vi "Filter Control Drop Event.vi"(8 "error in (no error)":errorcluster, 10 "ControlDropMsg":refnum<class "ControlDropMsg.lvclass">, 11 "Test Executive Builder Event Filter in":refnum<class "Test Executive Builder Event Filter.lvclass">) -> (0 "error out":errorcluster, 1 "Discard?":bool, 3 "Test Executive Builder Event Filter out":refnum<class "Test Executive Builder Event Filter.lvclass">)   [LabVIEW 2017, in "Test Executive Builder Event Filter.lvclass"]
uses:
  Test Executive Builder Event Filter.lvclass
  <vilib>/gpm_packages/@cs/mva-viewable/Source/ActorEvents/IEventAggregator Messages/ControlDropMsg/ControlDropMsg.lvclass
  Test Executive Builder View Messages/Handle Drop Msg/Handle Drop Msg.lvclass
  <vilib>/gpm_packages/@cs/actor-framework-messages/Source/RoundTripMessage/RoundTripMessage.lvclass
  C:/Users/jonmc/Documents/Git/Test Executive Builder/gpm_packages/@cs/actor-framework-messages/Source/RoundTripMessage/RoundTripMessage.lvclass
panel:
  # "No additional\nEvent Data"
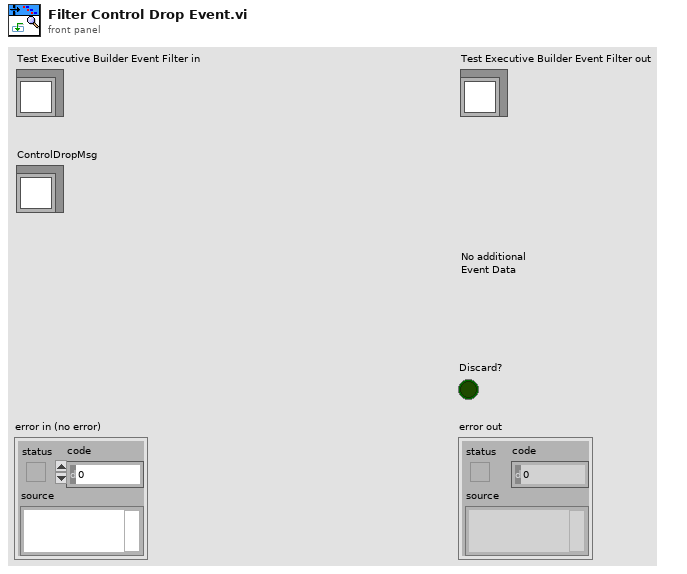
[diagram p1: front panel]
types:
  T1 = typedef "LVPoint32TypeDef.ctl" = cluster{"Horizontal":i32, "Vertical":i32}
  T2 = cluster{"Shift":bool, "Ctrl":bool, "Alt":bool, "Cmd":bool, "Opt":bool}
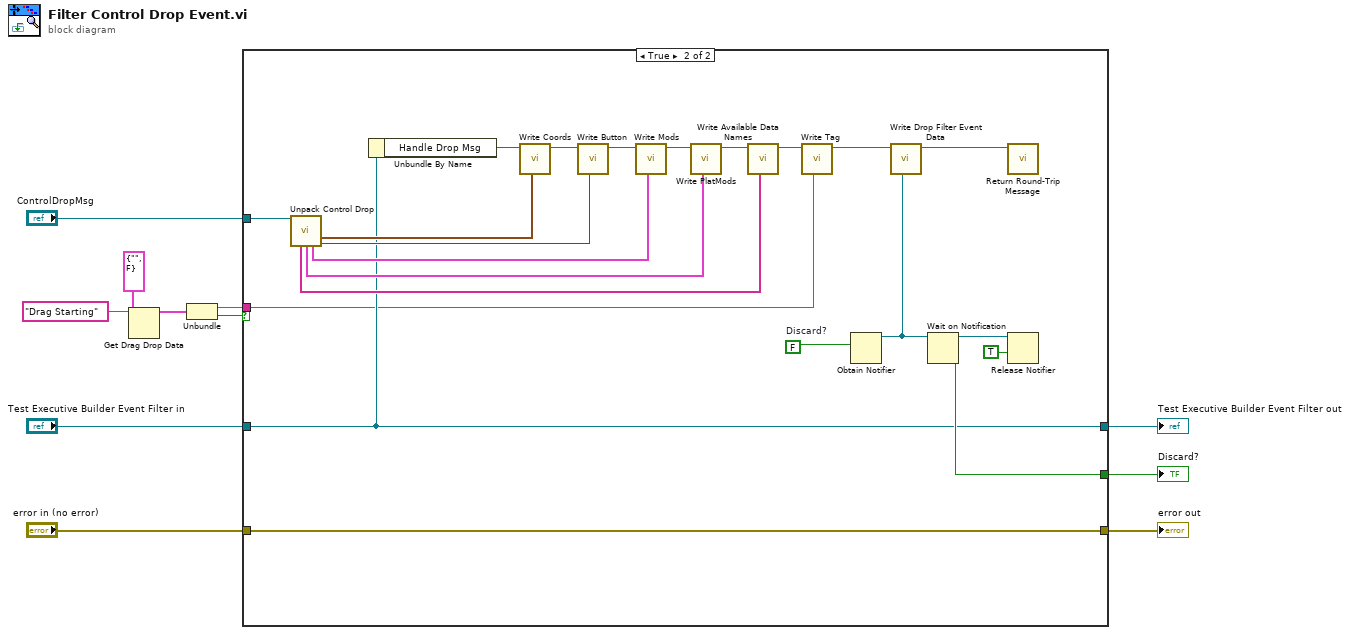
[diagram p0: block diagram]
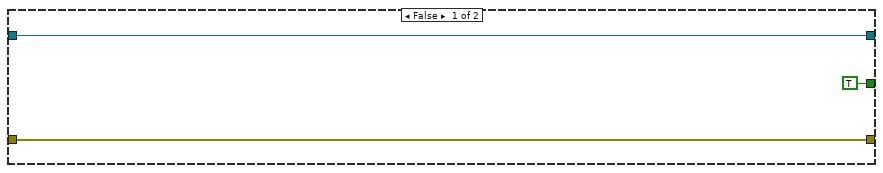
[diagram p2: hidden frame]
diagram:
  n1 = Get Drag Drop Data(8:cluster{"Tag":string, bool} {"Tag"="", FALSE}, 9:"Drag Starting" ("data name")) -> (3:w6:cluster{"Tag":string, bool})  [unwired: 1 in, 1 out]
  n2 = Unbundle(w6) -> ("Tag"=w1:string, w2:bool)
  n3 = case shown="True" w2 {
    tunnel: "ControlDropMsg" -> [_ w36]
    tunnel: [TRUE ("Discard?") w32] -> w10
    tunnel: "Test Executive Builder Event Filter in" -> [w14 w20]
    tunnel: [w14 w20] -> w5
    tunnel: [w12 w19] -> w4
    tunnel: "error in (no error)" -> [w12 w19]
    tunnel: w1 -> [_ w16]
    frame False {
    }
    frame True {
      w34 = FALSE  # Discard?
      n4 = call <vilib>:"Unpack Control Drop.vi"("ControlDropMsg"=w36) -> ("Coords"=w30:T1, "Available Data Names"=w22:string[], "PlatMods"=w24:T2, "Mods"=w26:cluster{"Double Click":bool, "Menu Key":bool}, "Button"=w28:u16)  [unwired: 7 in, 3 out]
      n5 = Unbundle By Name(w20) -> ("Handle Drop Msg"=w31:refnum<class "Handle Drop Msg.lvclass">)
      n6 = call "Write Coords.vi"("Coordinates"=w30, "Handle Drop Msg in"=w31) -> ("Handle Drop Msg out"=w29:refnum<class "Handle Drop Msg.lvclass">)  [unwired: 9 in]
      n7 = call "Write Button.vi"("Button"=w28, "Handle Drop Msg in"=w29) -> ("Handle Drop Msg out"=w27:refnum<class "Handle Drop Msg.lvclass">)  [unwired: 9 in]
      n8 = call "Write Mods.vi"("Mods"=w26, "Handle Drop Msg in"=w27) -> ("Handle Drop Msg out"=w25:refnum<class "Handle Drop Msg.lvclass">)  [unwired: 9 in]
      n9 = call "Write PlatMods.vi"("PlatMods"=w24, "Handle Drop Msg in"=w25) -> ("Handle Drop Msg out"=w23:refnum<class "Handle Drop Msg.lvclass">)  [unwired: 9 in]
      n10 = call "Write Available Data Names.vi"("Available Data Names"=w22, "Handle Drop Msg in"=w23) -> ("Handle Drop Msg out"=w18:refnum<class "Handle Drop Msg.lvclass">)  [unwired: 9 in]
      n11 = call "Write Tag.vi"("Tag"=w16, "Handle Drop Msg in"=w18) -> ("Handle Drop Msg out"=w17:refnum<class "Handle Drop Msg.lvclass">)  [unwired: 9 in]
      n12 = Obtain Notifier(notification data type=w34) -> (notifier out=w21:refnum<notifier>)  [unwired: 3 in, 2 out]
      n13 = call "Write Drop Filter Event Data.vi"("Drop Filter Event Data"=w21, "Handle Drop Msg in"=w17) -> ("Handle Drop Msg out"=w15:refnum<class "Handle Drop Msg.lvclass">)  [unwired: 9 in]
      n14 = Wait on Notification(notifier=w21) -> (notifier out=w33:refnum<notifier>, notification=w32:bool)  [unwired: 3 in, 2 out]
      n15 = call <vilib>:"Return Round-Trip Message.vi"("RoundTripMessage In"=w15) -> ()  [unwired: 10 in, 1 out]
      n16 = Release Notifier(notifier=w33, force destroy? (F)=TRUE) -> ()  [unwired: 1 in, 3 out]
    }
  }
  "error out" <- w4
  "Test Executive Builder Event Filter out" <- w5
  "Discard?" <- w10
